vi "Write Tab Dimension.vi"(5 "Tab Dimension":T1, 9 "Tab in":refnum<class "Tab.lvclass">) -> (3 "Tab out":refnum<class "Tab.lvclass">)   [LabVIEW 2014, in "Raspberry Pi Compatible Compiler for LabVIEW.lvlib" / "Tab.lvclass"]
uses:
  Tab.lvclass
  <vilib>/Utility/miscctls.llb/LVPointTypeDef.ctl
  Tab.lvclass/Tab.ctl
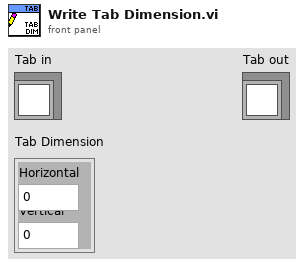
[diagram p1: front panel]
types:
  T1 = typedef "LVPointTypeDef.ctl" = cluster{"Horizontal":i16, "Vertical":i16}
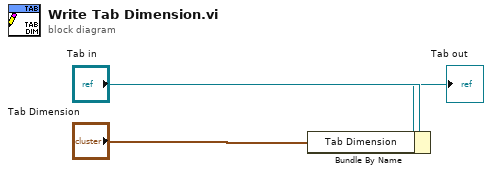
[diagram p0: block diagram]
diagram:
  n1 = Bundle By Name(cluster="Tab in", "Tab Dimension"="Tab Dimension") -> (→"Tab out":refnum<class "Tab.lvclass">)
